vi "Handle Routing Channel State Change.vi"(4 "force update":bool, 6 "init index":bool=TRUE, 7 "Alias Mappings":T1[](array[typedef]), 8 "error in (no error)":errorcluster, 9 "State":string, 10 "Routing Channel Page Controls":T2, 11 "Routing Channel Ref in":T3 format="%.0x") -> (0 "error out":errorcluster, 3 "Routing Channel Ref out":T3 format="%.0x")   [LabVIEW 2017, in "Routing and Faulting System Explorer.lvlib"]
uses:
  Routing and Faulting System Explorer.lvlib
  <vilib>/NI Veristand/Custom Device API/Custom Device Item Ref.ctl
  Routing Channel Page Controls.ctl
  Shared/Alias Mapping.ctl
  Scripting/Routing and Faulting Scripting.lvlib
  <vilib>/NI VeriStand/Custom Device API/Custom Device API.lvlib
  Shared/Routing and Faulting Shared.lvlib
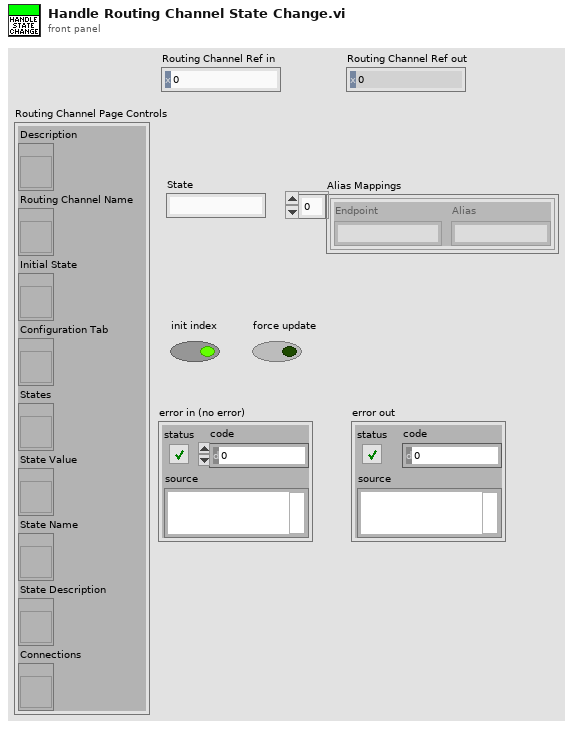
[diagram p1: front panel]
types:
  T1 = typedef "Routing and Faulting Shared.lvlib/Alias Mapping.ctl" = cluster{"Endpoint":string, "Alias":string}
  T2 = typedef "Routing and Faulting System Explorer.lvlib/Routing Channel Page Controls.ctl" = cluster{"Description":refnum<vi>, "Routing Channel Name":refnum<vi>, "Initial State":refnum<vi>, "Configuration Tab":refnum<vi>, "States":refnum<vi>, "State Value":refnum<vi>, "State Name":refnum<vi>, "State Description":refnum<vi>, "Connections":refnum<vi>}
  T3 = typedef "Custom Device API.lvlib/Custom Device Item Ref.ctl" = u64
  T4 = typedef "Routing and Faulting Shared.lvlib/Routing State.ctl" = cluster{"Name":string, "Description":string, "Value":i32, "Connection List":T5[]}
  T5 = typedef "Routing and Faulting Shared.lvlib/Connection.ctl" = cluster{"Module":string, "Source":string, "Destination":string}
  T6 = typedef "Routing and Faulting System Explorer.lvlib/State-Value Row.ctl" = cluster{"State":string, "State Value":string}
  T7 = typedef "Routing and Faulting System Explorer.lvlib/Connection Row.ctl" = cluster{"Source":string, "Destination":string, "Edit":bool, "Remove":bool}
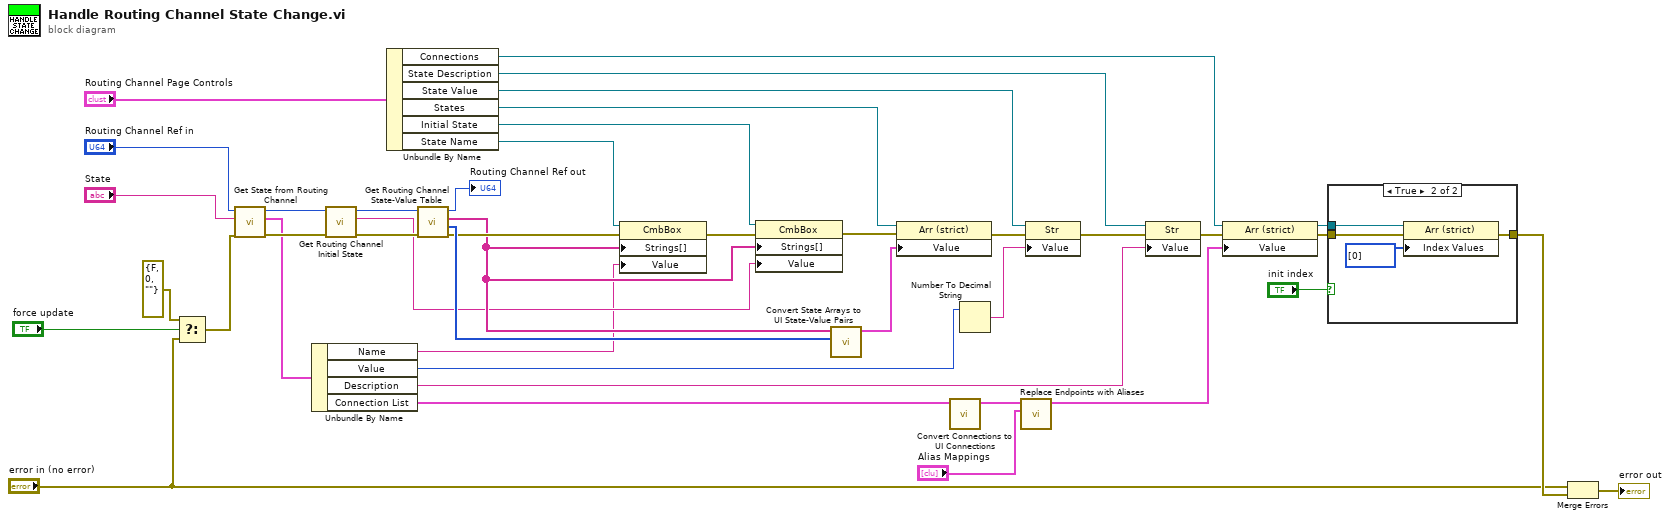
[diagram p0: block diagram]
diagram:
  n1 = Select(t=errorcluster {"status"=FALSE, "code"=0, "source"=""}, s="force update", f="error in (no error)") -> (s? t:f=w14:errorcluster)
  n2 = call "Get State from Routing Channel.vi"("error in (no error)"=w14, "State"="State", "Channel Ref in"="Routing Channel Ref in") -> ("error out"=w29:errorcluster, "State and Connections"=w26:T4, "Channel Ref out"=w9:T3)  [unwired: 6 in]
  n3 = Unbundle By Name(w26) -> ("Name"=w1:string, "Value"=w42:i32, "Description"=w36:string, "Connection List"=w39:T5[])
  n4 = call "Get Routing Channel Initial State.vi"("error in (no error)"=w29, "Channel Ref in"=w9) -> ("error out"=w10:errorcluster, "Initial State"=w6:string, "Channel Ref out"=w8:T3)  [unwired: 7 in]
  n5 = Unbundle By Name("Routing Channel Page Controls") -> ("Connections"=w20:refnum<vi>, "State Description"=w35:refnum<vi>, "State Value"=w2:refnum<vi>, "States"=w23:refnum<vi>, "Initial State"=w5:refnum<vi>, "State Name"=w22:refnum<vi>)
  n6 = call "Get Routing Channel State-Value Table.vi"("error in (no error)"=w10, "Channel Ref in"=w8) -> ("error out"=w25:errorcluster, "State Values"=w28:i32[], "State Names"=w7:string[], "Channel Ref out"=→"Routing Channel Ref out":T3)  [unwired: 6 in]
  n7 = property class="CmbBox"(reference=w22, error in=w25, "Strings[]"=w7, "Value"=w1) -> (error out=w4:errorcluster)  [unwired: 1 out]
  n8 = property class="CmbBox"(reference=w5, error in=w4, "Strings[]"=w7, "Value"=w6) -> (error out=w3:errorcluster)  [unwired: 1 out]
  n9 = call "Convert State Arrays to UI State-Value Pairs.vi"("State Values"=w28, "State Names"=w7) -> ("State-Value Pairs"=w27:T6[])  [unwired: 9 in]
  n10 = property class="Arr (strict)"(reference=w23, error in=w3, "Value"=w27) -> (error out=w24:errorcluster)  [unwired: 1 out]
  n11 = call "Convert Connections to UI Connections.vi"("Connection List"=w39) -> ("UI Connections List"=w33:T7[])  [unwired: 10 in]
  n12 = Number To Decimal String(number=w42) -> (decimal integer string=w21:string)  [unwired: 1 in]
  n13 = call "Replace Endpoints with Aliases.vi"("Alias Mappings"="Alias Mappings", "UI Connections List in"=w33) -> ("UI Connections List out"=w32:T7[])  [unwired: 9 in]
  n14 = property class="Str"(reference=w2, error in=w24, "Value"=w21) -> (error out=w38:errorcluster)  [unwired: 1 out]
  n15 = property class="Str"(reference=w35, error in=w38, "Value"=w36) -> (error out=w37:errorcluster)  [unwired: 1 out]
  n16 = property class="Arr (strict)"(reference=w20, error in=w37, "Value"=w32) -> (reference out=w19:refnum<vi>, error out=w18:errorcluster)
  n17 = case shown="True" "init index" {
    tunnel: w19 -> [_ w46]
    tunnel: w18 -> [w43 w45]
    tunnel: [w43 w44] -> w13
    frame False {
    }
    frame True {
      n18 = property class="Arr (strict)"(reference=w46, error in=w45, "Index Values"=u32[] [0]) -> (error out=w44:errorcluster)  [unwired: 1 out]
    }
  }
  n19 = Merge Errors("error in (no error)", w13) -> (→"error out":errorcluster)
